vi "create Behaviour.vi"(8 "error in (no error)":errorcluster caption="Fehler (Eingang, kein Fehler)", 11 "Surge Eingang":refnum<class "Surge.lvclass"> caption="DNL_LabVIEW Object in") -> (0 "error out":errorcluster caption="Fehler (Ausgang)", 1 "regex":string[](array[string]), 2 "response":bool[](array[boolean]), 3 "Surge Ausgang":refnum<class "Surge.lvclass"> caption="DNL_LabVIEW Object out")   [LabVIEW 2013, in "Surge.lvclass"]
uses:
  Surge.lvclass
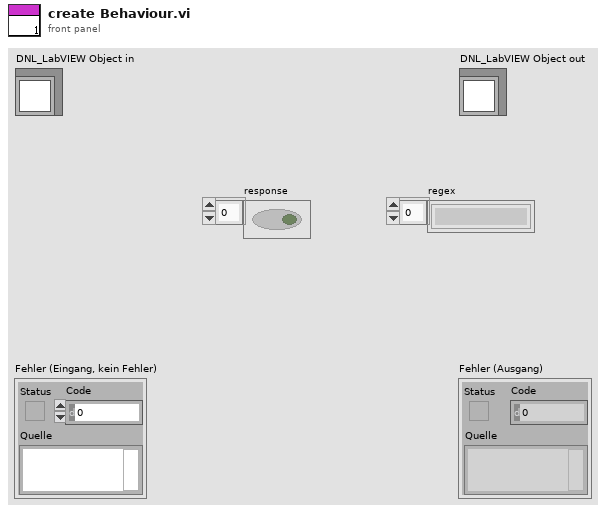
[diagram p1: front panel]
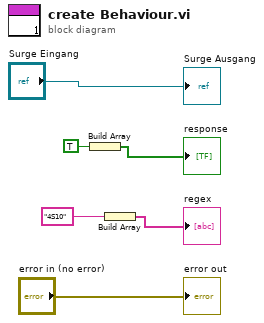
[diagram p0: block diagram]
diagram:
  n1 = Build Array(TRUE) -> (→"response":bool[])
  n2 = Build Array("4S10") -> (→"regex":string[])
  "error out" <- "error in (no error)"
  "Surge Ausgang" <- "Surge Eingang"
